vi "Col_32B_v2.vi"(9 "Ref":dbl=300000.0 format="%#_13g", 11 "Col":dbl) -> (0 "LL":u8, 1 "LH":u8, 2 "HL":u8, 3 "HH":u8)   [LabVIEW 2017]
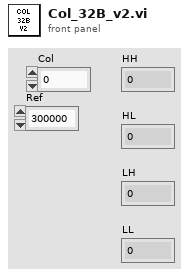
[diagram p1: front panel]
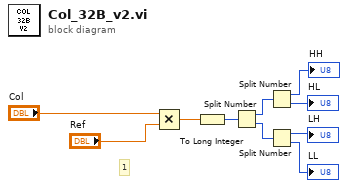
[diagram p0: block diagram]
diagram:
  # "1"
  n1 = Multiply(x="Col", y="Ref") -> (x*y=w5:dbl)
  n2 = To Long Integer(number=w5) -> (32bit integer=w1:i32)
  n3 = Split Number(x=w1) -> (hi(x)=w3:u16, lo(x)=w2:u16)
  n4 = Split Number(x=w3) -> (hi(x)=→"HH":u8, lo(x)=→"HL":u8)
  n5 = Split Number(x=w2) -> (hi(x)=→"LH":u8, lo(x)=→"LL":u8)
